vi "parseBMSPdo.vi"(8 "error in (no error)":errorcluster, 9 "PDO channel":u8(ring) items=["PDO 1", "PDO 2", "PDO 3", "PDO 4"], 10 "TPDO data":u8[](array[numeric]) format="%x", 11 "Orion_BMS in":refnum<class "Orion_BMS.lvclass">) -> (0 "error out":errorcluster, 3 "Orion_BMS out":refnum<class "Orion_BMS.lvclass">)   [LabVIEW 2018, in "Orion_BMS.lvclass"]
uses:
  Orion_BMS.lvclass
  Orion_BMS.lvclass/Orion_BMS.ctl
  <vilib>/CANopenLib/CANOPEN.llb/CANopen Fetch from Data [U16].vi
  <vilib>/CANopenLib/CANOPEN.llb/CANopen Fetch from Data [I8].vi
  <vilib>/CANopenLib/CANOPEN.llb/CANopen Fetch from Data [I16].vi
  <vilib>/CANopenLib/CANOPEN.llb/CANopen Fetch from Data [U8].vi
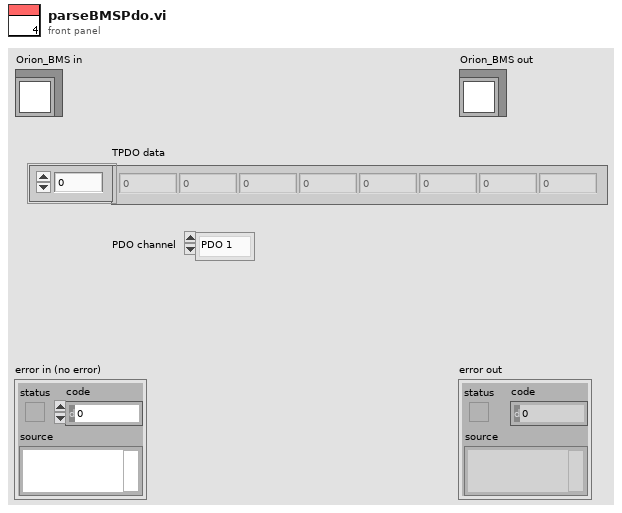
[diagram p1: front panel]
types:
  T1 = typedef "TypeDef_BMSData.ctl" = cluster{"Max Cell Voltage (V)":dbl, "Max Cell ID":dbl, "Min Cell Voltage (V)":dbl, "Min Cell ID":dbl, "State of Charge (%)":dbl, "Average Voltage (V)":dbl, "Voltage Delta (V)":dbl, "Pack Current (A)":dbl, "Pack Voltage (V)":dbl, "Max Resistance (Ohm)":dbl, "Min Resistance (Ohm)":dbl, "Average Resistance (Ohm)":dbl, "Delta Resistance (Ohm)":dbl, "Highest Temperature(F)":dbl, "BmsStatus":T2}
  T2 = typedef "TypeDef_BMS_Status.ctl" = cluster{"isFault":bool, "isolationMonitoring":bool}
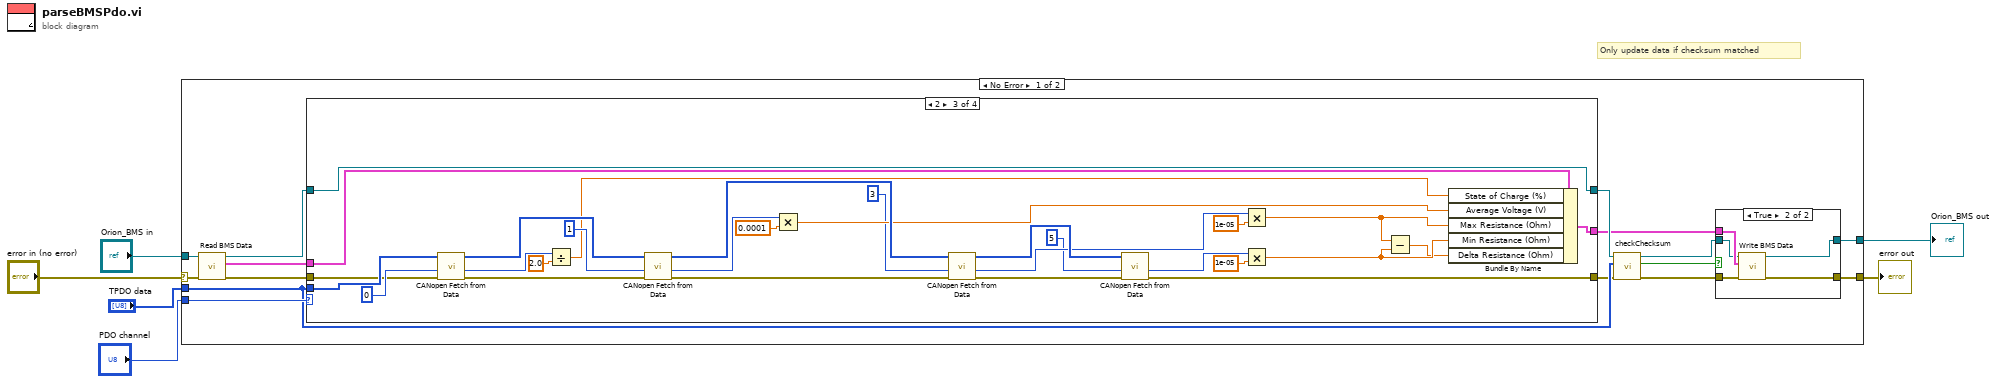
[diagram p0: block diagram]
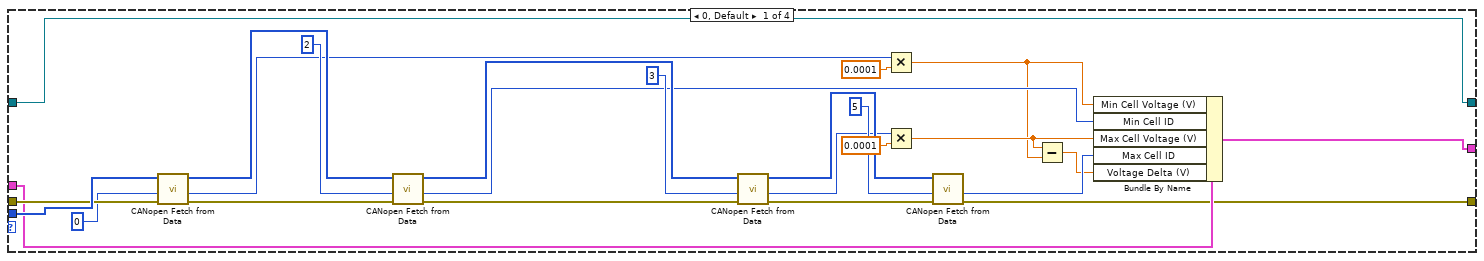
[diagram p3: hidden frame]
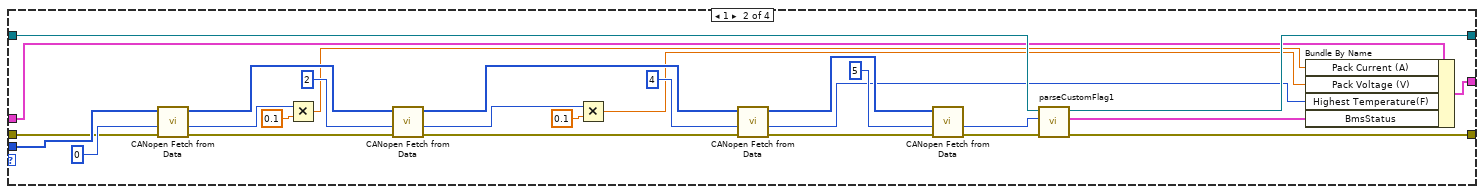
[diagram p4: hidden frame]
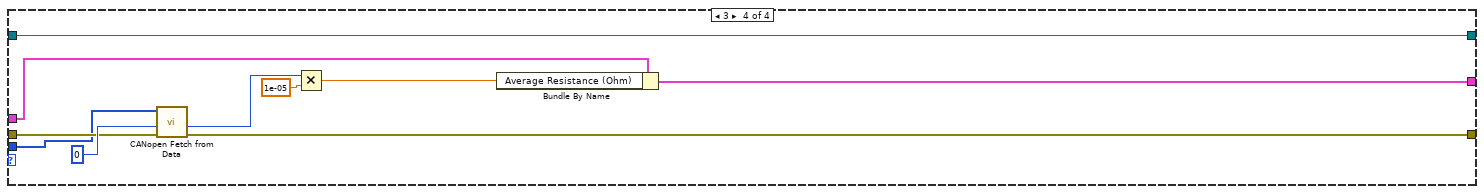
[diagram p5: hidden frame]
diagram:
  # "Only update data if checksum matched"
  n1 = case shown="No Error" "error in (no error)" {
    selector: "error in (no error)" -> [w19 w121]
    tunnel: [w8 w121] -> w1
    tunnel: "Orion_BMS in" -> [w20 w120]
    tunnel: "PDO channel" -> [w21 _]
    tunnel: "TPDO data" -> [w14 _]
    tunnel: [w11 w120] -> w2
    frame No Error {
      n2 = call "Read BMS Data.vi"("error in (no error)"=w19, "Orion_BMS in"=w20) -> ("error out"=w18:errorcluster, "BMS Data"=w17:T1, "Orion_BMS out"=w16:refnum<class "Orion_BMS.lvclass">)  [unwired: 7 in]
      n3 = case shown="2" w21 {
        tunnel: w14 -> [w53 w67 w109 w116]
        tunnel: w18 -> [w52 w66 w107 w117]
        tunnel: w17 -> [w39 w61 w102 w115]
        tunnel: [w33 w56 w87 w110] -> w12
        tunnel: w16 -> [w34 w64 w106 w119]
        tunnel: [w32 w63 w86 w114] -> w13
        tunnel: [w34 w62 w106 w119] -> w15
        frame 0, Default {
          n4 = call-poly <vilib>:"CANopen Fetch from Data.vi"("error in (no error)"=w52, "offset (0)"=u32 0, "CANopen data in"=w53) -> ("error out"=w47:errorcluster, "unsigned 16-bit integer"=w40:u16, "CANopen data out"=w51:u8[])  [unwired: 6 in]
          n5 = call-poly <vilib>:"CANopen Fetch from Data.vi"("error in (no error)"=w47, "offset (0)"=u32 2, "CANopen data in"=w51) -> ("error out"=w46:errorcluster, "signed 8-bit integer"=w38:i8, "CANopen data out"=w42:u8[])  [unwired: 6 in]
          n6 = call-poly <vilib>:"CANopen Fetch from Data.vi"("error in (no error)"=w46, "offset (0)"=u32 3, "CANopen data in"=w42) -> ("error out"=w45:errorcluster, "unsigned 16-bit integer"=w37:u16, "CANopen data out"=w43:u8[])  [unwired: 6 in]
          n7 = Multiply(x=w40, y=0.0001) -> (x*y=w30:dbl)
          n8 = Multiply(x=w37, y=0.0001) -> (x*y=w31:dbl)
          n9 = call-poly <vilib>:"CANopen Fetch from Data.vi"("error in (no error)"=w45, "offset (0)"=u32 5, "CANopen data in"=w43) -> ("error out"=w32:errorcluster, "signed 8-bit integer"=w35:i8)  [unwired: 6 in, 1 out]
          n10 = Subtract(x=w31, y=w30) -> (x-y=w29:dbl)
          n11 = Bundle By Name(cluster=w39, "Min Cell Voltage (V)"=w30, "Min Cell ID"=w38, "Max Cell Voltage (V)"=w31, "Max Cell ID"=w35, "Voltage Delta (V)"=w29) -> (w33:T1)
        }
        frame 1 {
          n12 = call-poly <vilib>:"CANopen Fetch from Data.vi"("error in (no error)"=w66, "offset (0)"=u32 0, "CANopen data in"=w67) -> ("error out"=w76:errorcluster, "unsigned 16-bit integer"=w69:u16, "CANopen data out"=w80:u8[])  [unwired: 6 in]
          n13 = Multiply(x=w69, y=0.1) -> (x*y=w60:dbl)
          n14 = call-poly <vilib>:"CANopen Fetch from Data.vi"("error in (no error)"=w76, "offset (0)"=u32 2, "CANopen data in"=w80) -> ("error out"=w75:errorcluster, "signed 16-bit integer"=w65:i16, "CANopen data out"=w71:u8[])  [unwired: 6 in]
          n15 = Multiply(x=w65, y=0.1) -> (x*y=w59:dbl)
          n16 = call-poly <vilib>:"CANopen Fetch from Data.vi"("error in (no error)"=w75, "offset (0)"=u32 4, "CANopen data in"=w71) -> ("error out"=w74:errorcluster, "signed 8-bit integer"=w58:i8, "CANopen data out"=w72:u8[])  [unwired: 6 in]
          n17 = call-poly <vilib>:"CANopen Fetch from Data.vi"("error in (no error)"=w74, "offset (0)"=u32 5, "CANopen data in"=w72) -> ("error out"=w55:errorcluster, "signed 8-bit integer"=w54:i8)  [unwired: 6 in, 1 out]
          n18 = call "parseCustomFlag1.vi"("error in (no error)"=w55, "Numeric"=w54, "Orion_BMS in"=w64) -> ("error out"=w63:errorcluster, "output cluster"=w57:T2, "Orion_BMS out"=w62:refnum<class "Orion_BMS.lvclass">)  [unwired: 6 in]
          n19 = Bundle By Name(cluster=w61, "Pack Current (A)"=w60, "Pack Voltage (V)"=w59, "Highest Temperature(F)"=w58, "BmsStatus"=w57) -> (w56:T1)
        }
        frame 2 {
          n20 = call-poly <vilib>:"CANopen Fetch from Data.vi"("error in (no error)"=w107, "offset (0)"=u32 0, "CANopen data in"=w109) -> ("error out"=w101:errorcluster, "unsigned 8-bit integer"=w83:u8, "CANopen data out"=w105:u8[])  [unwired: 6 in]
          n21 = Divide(x=w83, y=2.0) -> (x/y=w82:dbl)
          n22 = call-poly <vilib>:"CANopen Fetch from Data.vi"("error in (no error)"=w101, "offset (0)"=u32 1, "CANopen data in"=w105) -> ("error out"=w100:errorcluster, "unsigned 16-bit integer"=w97:u16, "CANopen data out"=w104:u8[])  [unwired: 6 in]
          n23 = Multiply(x=w97, y=0.0001) -> (x*y=w95:dbl)
          n24 = call-poly <vilib>:"CANopen Fetch from Data.vi"("error in (no error)"=w100, "offset (0)"=u32 3, "CANopen data in"=w104) -> ("error out"=w99:errorcluster, "unsigned 16-bit integer"=w93:u16, "CANopen data out"=w103:u8[])  [unwired: 6 in]
          n25 = call-poly <vilib>:"CANopen Fetch from Data.vi"("error in (no error)"=w99, "offset (0)"=u32 5, "CANopen data in"=w103) -> ("error out"=w86:errorcluster, "unsigned 16-bit integer"=w91:u16)  [unwired: 6 in, 1 out]
          n26 = Multiply(x=w93, y=1e-05) -> (x*y=w90:dbl)
          n27 = Multiply(x=w91, y=1e-05) -> (x*y=w89:dbl)
          n28 = Subtract(x=w90, y=w89) -> (x-y=w88:dbl)
          n29 = Bundle By Name(cluster=w102, "State of Charge (%)"=w82, "Average Voltage (V)"=w95, "Max Resistance (Ohm)"=w90, "Min Resistance (Ohm)"=w89, "Delta Resistance (Ohm)"=w88) -> (w87:T1)
        }
        frame 3 {
          n30 = call-poly <vilib>:"CANopen Fetch from Data.vi"("error in (no error)"=w117, "offset (0)"=u32 0, "CANopen data in"=w116) -> ("error out"=w114:errorcluster, "signed 16-bit integer"=w112:i16)  [unwired: 6 in, 1 out]
          n31 = Multiply(x=w112, y=1e-05) -> (x*y=w111:dbl)
          n32 = Bundle By Name(cluster=w115, "Average Resistance (Ohm)"=w111) -> (w110:T1)
        }
      }
      n33 = call "checkChecksum.vi"("error in (no error)"=w13, "TPDO data"=w14, "Orion_BMS in"=w15) -> ("error out"=w9:errorcluster, "checkSumMatched"=w10:bool, "Orion_BMS out"=w7:refnum<class "Orion_BMS.lvclass">)  [unwired: 6 in]
      n34 = case shown="True" w10 {
        tunnel: w12 -> [_ w28]
        tunnel: [w23 w27] -> w11
        tunnel: w9 -> [w22 w26]
        tunnel: [w22 w25] -> w8
        tunnel: w7 -> [w23 w24]
        frame False {
        }
        frame True {
          n35 = call "Write BMS Data.vi"("error in (no error)"=w26, "BMS Data"=w28, "Orion_BMS in"=w24) -> ("error out"=w25:errorcluster, "Orion_BMS out"=w27:refnum<class "Orion_BMS.lvclass">)  [unwired: 7 in]
        }
      }
    }
    frame Error {
    }
  }
  "error out" <- w1
  "Orion_BMS out" <- w2
